vi "LoadLvClassInDir.vi"(8 "error in":errorcluster, 9 "options":u32, 11 "appended path":path) -> (0 "error out":errorcluster, 3 "Array":refnum<class>[](array[class]))   [LabVIEW 2014]
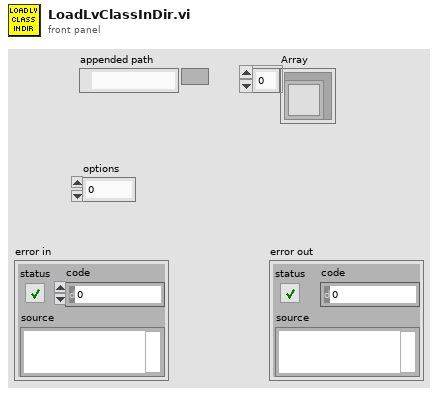
[diagram p1: front panel]
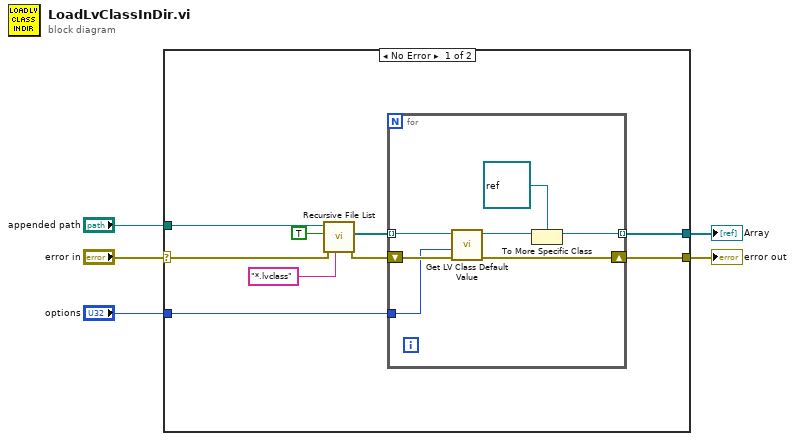
[diagram p0: block diagram]
diagram:
  n1 = case shown="No Error" "error in" {
    selector: "error in" -> [w6 w22]
    tunnel: [w14 _] -> w5
    tunnel: [w13 w22] -> w4
    tunnel: "options" -> [w12 _]
    tunnel: "appended path" -> [w7 _]
    frame No Error {
      n2 = call <vilib>:"Recursive File List.vi"("pattern"="*.lvclass", "error in (no error)"=w6, "Treat LLBs as Folders?"=TRUE, "Folder Path"=w7) -> ("error out"=w11:errorcluster, "All Files in Dir"=w10:path[])  [unwired: 3 in, 3 out]
      n3 = for {
        tunnel: w10 -> [w21] mode=indexing
        shift-right: [w18] -> w13
        shift-left: w11 -> [w20]
        tunnel: w12 -> [w17]
        tunnel: [w16] -> w14 mode=indexing
        n4 = call <vilib>:"Get LV Class Default Value.vi"("error in (no error)"=w20, "options"=w17, "class path"=w21) -> ("error out"=w18:errorcluster, "object"=w19:refnum<class>)  [unwired: 7 in]
        n5 = To More Specific Class(target class=refnum<class> refnum ("LabVIEW Object"), reference=w19) -> (specific class reference=w16:refnum<class>)  [unwired: 1 in, 1 out]
      }
    }
    frame Error {
    }
  }
  "Array" <- w5
  "error out" <- w4
